vi "removeNode.vi"(8 "error in (no error)":errorcluster, 10 "Node Path":string, 11 "xceRootNode in":refnum<class "xceRootNode.lvclass">) -> (0 "error out":errorcluster, 3 "xceRootNode out":refnum<class "xceRootNode.lvclass">)   [LabVIEW 2013, in "xceRootNode.lvclass"]
doc: "Removes a node from the tree data structure, and the tree control."
uses:
  xceRootNode.lvclass
  xceNode/xceNode.lvclass
  xceRootNode.lvclass/xceRootNode.ctl
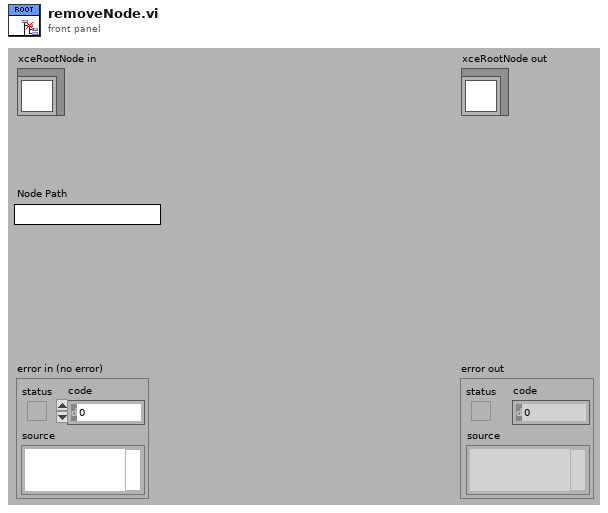
[diagram p1: front panel]
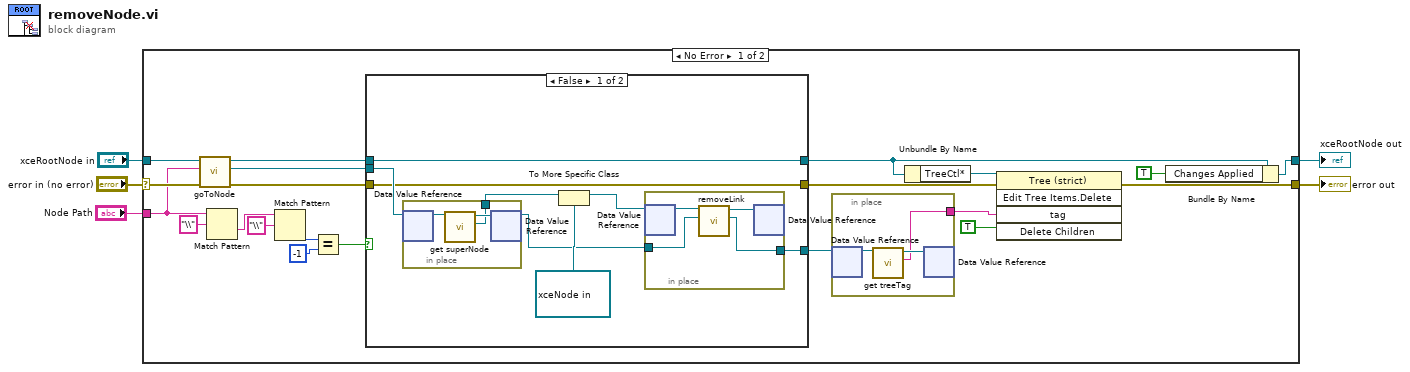
[diagram p0: block diagram]
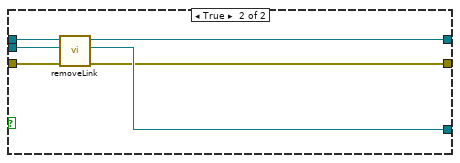
[diagram p2: hidden frame]
diagram:
  n1 = case shown="No Error" "error in (no error)" {
    selector: "error in (no error)" -> [w25 w52]
    tunnel: [w9 w52] -> w4
    tunnel: [w7 w51] -> w2
    tunnel: "xceRootNode in" -> [w26 w51]
    tunnel: "Node Path" -> [w24 _]
    frame No Error {
      n2 = call "goToNode.vi"("error in (no error)"=w25, "Node Path"=w24, "xceNode in"=w26) -> ("error out"=w17:errorcluster, "goToNode* out"=w16:refnum<data-value>, "xceNode out"=w14:refnum<class "xceRootNode.lvclass">)  [unwired: 6 in]
      n3 = Match Pattern(string=w24, regular expression="\\") -> (after substring=w21:string)  [unwired: 1 in, 3 out]
      n4 = Match Pattern(string=w21, regular expression="\\") -> (offset past match=w20:i32)  [unwired: 1 in, 3 out]
      n5 = Equal?(x=w20, y=-1) -> (x = y?=w18:bool)
      n6 = case shown="False" w18 {
        tunnel: w14 -> [w31 w46]
        tunnel: w17 -> [w30 w48]
        tunnel: w16 -> [w37 w50]
        tunnel: [w32 w49] -> w15
        tunnel: [w31 w47] -> w8
        tunnel: [w30 w45] -> w10
        frame False {
          n7 = in-place {
            in-place-border: [w42] -> w36
            n8 = in-place-dvr #1(w37) -> (w44:refnum<class "xceNode.lvclass">)  [unwired: 1 out]
            n9 = call "get superNode.vi"("xceNode in"=w44) -> ("superNode*"=w42:refnum<data-value>, "xceNode out"=w43:refnum<class "xceNode.lvclass">)  [unwired: 8 in, 1 out]
            n10 = in-place-dvr #1(w43) -> (w33:refnum<data-value>)  [unwired: 1 out]
          }
          n11 = To More Specific Class(target class=refnum<data-value> refnum ("goToNode* out"), reference=w36) -> (specific class reference=w35:refnum<data-value>)  [unwired: 1 in, 1 out]
          n12 = in-place {
            in-place-border: w33 -> [w40]
            in-place-border: [w38] -> w32
            n13 = in-place-dvr #2(w35) -> (w41:refnum<class "xceNode.lvclass">)  [unwired: 1 out]
            n14 = call "removeLink.vi"("subNode in"=w40, "superNode in"=w41) -> ("subNode out"=w38:refnum<data-value>, "superNode out"=w39:refnum<class "xceNode.lvclass">)  [unwired: 7 in, 1 out]
            n15 = in-place-dvr #2(w39) -> ()  [unwired: 2 out]
          }
        }
        frame True {
          n16 = call "removeLink.vi"("error in (no error)"=w48, "subNode in"=w50, "superNode in"=w46) -> ("error out"=w45:errorcluster, "subNode out"=w49:refnum<data-value>, "superNode out"=w47:refnum<class "xceRootNode.lvclass">)  [unwired: 6 in]
        }
      }
      n17 = in-place {
        in-place-border: [w27] -> w12
        n18 = in-place-dvr #3(w15) -> (w29:refnum<class "xceNode.lvclass">)  [unwired: 1 out]
        n19 = call "get treeTag.vi"("xceNode in"=w29) -> ("treeTag"=w27:string, "xceNode out"=w28:refnum<class "xceNode.lvclass">)  [unwired: 8 in, 1 out]
        n20 = in-place-dvr #3(w28) -> ()  [unwired: 2 out]
      }
      n21 = Unbundle By Name(w8) -> ("TreeCtl*"=w13:refnum<vi>)
      n22 = invoke class="Tree (strict)" method="Edit Tree Items.Delete"(reference=w13, error in=w10, "tag"=w12, "Delete Children"=TRUE ("Delete Children?")) -> (error out=w9:errorcluster)  [unwired: 1 in, 4 out]
      n23 = Bundle By Name(cluster=w8, "Changes Applied"=TRUE) -> (w7:refnum<class "xceRootNode.lvclass">)
    }
    frame Error {
    }
  }
  "error out" <- w4
  "xceRootNode out" <- w2
